vi "Write.vi"   [LabVIEW 2011]
uses:
  WS2812.lvlib
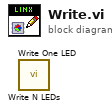
[diagram p0: block diagram]
diagram:
  n1 = call "Write N LEDs.vi"() -> ()  [unwired: 10 in, 2 out]
  n2 = call "Write One LED.vi"() -> ()  [unwired: 10 in, 2 out]
